vi "ImPro - Contrast Adjustment.vi"(8 "error in (no error)":errorcluster, 10 "24-bit pixmap In":u32[][](array[numeric]), 11 "Contrast":dbl) -> (0 "error out":errorcluster, 2 "24-bit pixmap Out":u32[][](array[numeric]))   [LabVIEW 2023]
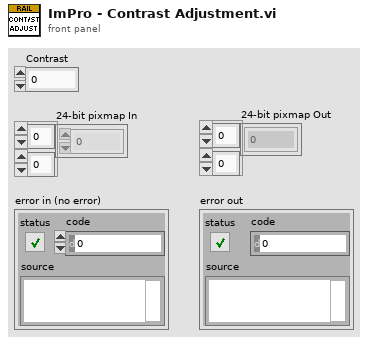
[diagram p1: front panel]
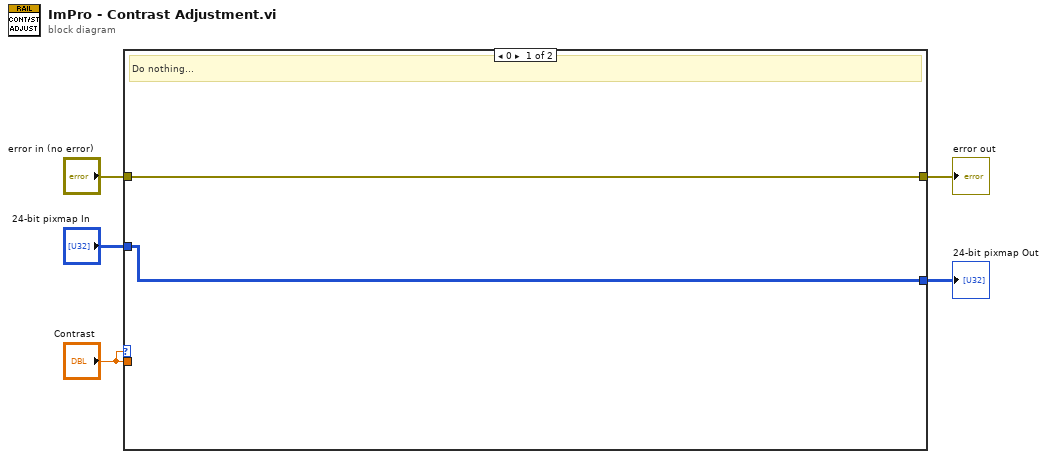
[diagram p0: block diagram]
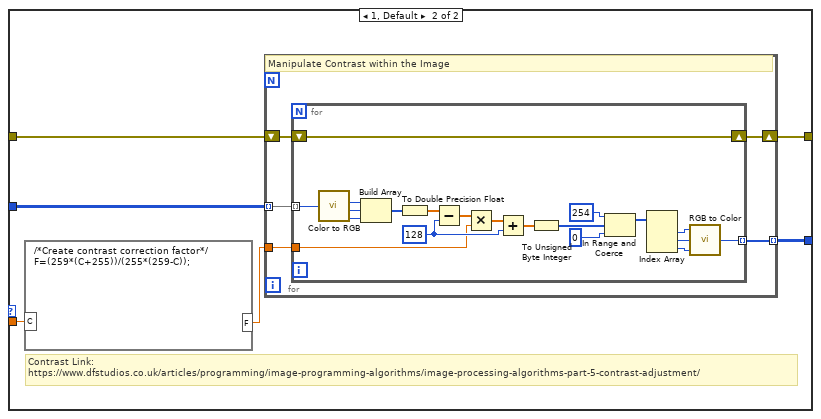
[diagram p2: hidden frame]
diagram:
  n1 = case shown="0" "Contrast" {
    tunnel: [w6 w13] -> w5
    tunnel: "error in (no error)" -> [w6 w12]
    tunnel: "Contrast" -> [_ w11]
    tunnel: "24-bit pixmap In" -> [w7 w10]
    tunnel: [w7 w9] -> w2
    frame 0 {
      # "Do nothing..."
    }
    frame 1, Default {
      # "Contrast Link:\nhttps://www.dfstudios.co.uk/articles/programming/image-programming-algorithms/image-processing-algorithms-part-5-contrast-adjustment/"
      n2 = formula code="/*Create contrast correction factor*/\nF=(259*(C+255))/(255*(259-C));"("C"=w11) -> ("F"=w8:dbl)
      n3 = for {
        tunnel: w10 -> [w18] mode=indexing
        tunnel: w8 -> [w17]
        tunnel: [w16] -> w9 mode=indexing
        shift-right: [w14] -> w13
        shift-left: w12 -> [w15]
        # "Manipulate Contrast within the Image"
        n4 = for {
          tunnel: w18 -> [w38] mode=indexing
          tunnel: w17 -> [w22]
          tunnel: [w30] -> w16 mode=indexing
          shift-right: [w19] -> w14
          shift-left: w15 -> [w19]
          w24 = u8 128 ("unsigned 8bit integer")
          n5 = call <vilib>:"Color to RGB.vi"("Color"=w38) -> ("R"=w28:u8, "G"=w37:u8, "B"=w36:u8)  [unwired: 1 out]
          n6 = Build Array(w28, w37, w36) -> (w27:u8[])
          n7 = To Double Precision Float(number=w27) -> (double precision float=w20:dbl[])
          n8 = Subtract(x=w20, y=w24) -> (x-y=w26:dbl[])
          n9 = Multiply(x=w26, y=w22) -> (x*y=w25:dbl[])
          n10 = Add(x=w25, y=w24) -> (x+y=w23:dbl[])
          n11 = To Unsigned Byte Integer(number=w23) -> (unsigned 8bit integer=w21:u8[])
          n12 = In Range and Coerce(upper limit=u8 254, x=w21, lower limit=u8 0) -> (coerced(x)=w33:u8[])  [unwired: 1 out]
          n13 = Index Array(array=w33) -> (element #1=w29:u8, element #2=w32:u8, element #3=w31:u8)  [unwired: 3 in]
          n14 = call <vilib>:"RGB to Color.vi"("B"=w31, "G"=w32, "R"=w29) -> ("Color"=w30:u32)
        }
      }
    }
  }
  "error out" <- w5
  "24-bit pixmap Out" <- w2
